vi "asdf.vi"(0 "ROI Descriptor (Image Mask 2)":T2={"Global Rectangle"=[63, 47, 555, 457], "Contours"=[{"ID"=enum."External", "Type"=3, "Coordinates"=[63, 47, 555, 457]}]} {"Contours"."Type" items=["No Selection", "Point", "Line", "Rectangle", "Oval", "Polygon", "Freehand Region", "Annulus", "Unused2", "Unused3", "Broken Line", "Freehand Line", "Rotated Rectangle"]}, 1 "Shrink (Image Mask 2)":bool=TRUE, 2 "Out / In (Image Mask 2)":bool, 3 "Color Plane (Color Plane Extraction 2)":i32(ring)=1 items=["Red", "Green", "Blue", "Hue", "Saturation", "Luminance", "Value", "Intensity"], 4 "Range (Threshold 3)":cluster{"Lower value":sgl, "Upper value":sgl}={"Lower value"=0.0, "Upper value"=222.0}, 5 "Operation (Gray Morphology 3)":T1(ring)=enum."Open", 6 "Structuring Element (Gray Morphology 3)":i32[][](array[numeric])=[[0, 1, 0], [1, 1, 1], [0, 1, 0]], 7 "error in":errorcluster, 8 "Min Radius (Circle Detection 2)":sgl=8.0, 9 "Max Radius (Circle Detection 2)":sgl=280.0) -> (20 "Nb Circles (Circle Detection 2)":i32, 21 "Circles Data (Circle Detection 2)":T4(array[cluster]), 22 "Circles Data (calibrated) (Circle Detection 2)":T4(array[cluster]), 27 "error out":errorcluster)   [LabVIEW 2018]
uses:
  <vilib>/vision/NI_Vision_Development_Module.lvlib
panel:
  out "Image Out":T3(plugin-control)
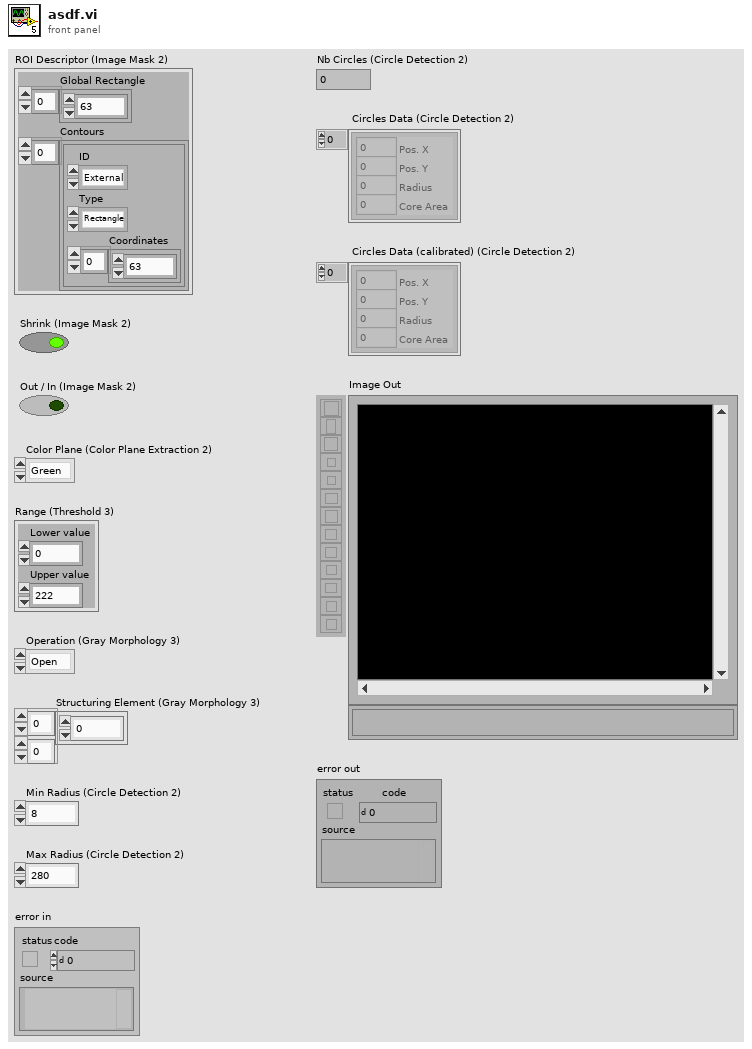
[diagram p1: front panel]
types:
  T1 = enum32{"AutoM", "Close", "Dilate", "Erode", "Gradient", "Gradient in", "Gradient out", "HitMiss", "Open", "PClose", "POpen", "Thick", "Thin"}
  T2 = cluster{"Global Rectangle":i32[], "Contours":cluster{"ID":enum32{"External", "Internal"}, "Type":u32, "Coordinates":i32[]}[]}
  T3 = typedef "IMAQ Image.ctl" = refnum<image>
  T4 = cluster{"Pos. X":i32, "Pos. Y":i32, "Radius":i32, "Core Area":i32}[]
  T5 = typedef "Image Type" = u32
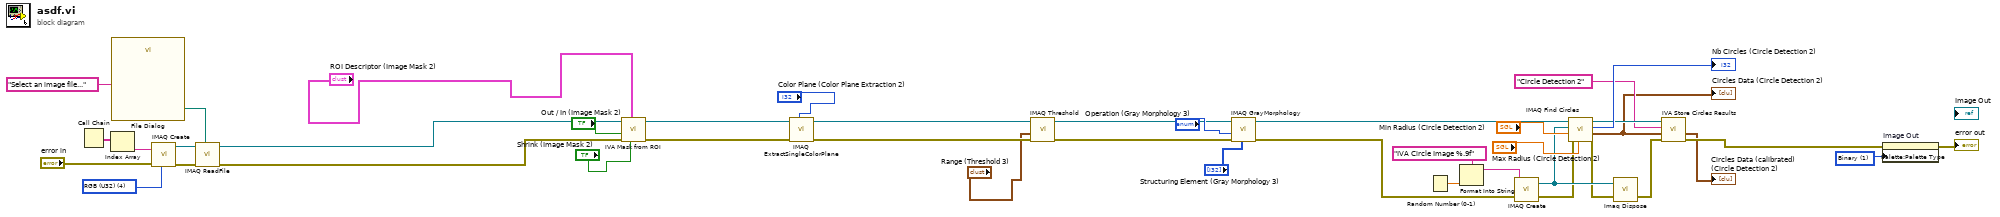
[diagram p0: block diagram]
diagram:
  w1 = u32 1 items=["Grayscale", "Binary", "Gradient", "Rainbow", "Temperature", "User Defined", "Binary 16 Bit", "Gradient 16 Bit", "Rainbow 16 Bit", "Temperature 16 Bit", "User Defined 16 Bit"] ("Palette Type")
  w33 = T5 4 items=["Grayscale (U8)", "Grayscale (I16)", "Grayscale (SGL)", "Complex (CSG)", "RGB (U32)", "HSL (U32)", "RGB (U64)", "Grayscale (U16)"] ("Image Type")
  n1 = Call Chain() -> (call chain=w37:string[])
  n2 = Index Array(array=w37) -> (element=w36:string)  [unwired: 1 in]
  n3 = call "File Dialog"("prompt"="Select an image file...") -> ("selected path"=w34:path)  [unwired: 6 in, 8 out]
  n4 = call "IMAQ Create"("Image Name"=w36, "Image Type"=w33, "error in (no error)"="error in") -> ("New Image"=w40:T3, "error out"=w39:errorcluster)  [unwired: 1 in, 1 out]
  n5 = call "IMAQ ReadFile"("File Path"=w34, "error in (no error)"=w39, "Image"=w40) -> ("error out"=w41:errorcluster, "Image Out"=w30:T3)  [unwired: 2 in, 5 out]
  n6 = call <vilib>:"IVA Mask from ROI.vi"("Shrink"="Shrink (Image Mask 2)", "ROI Descriptor"="ROI Descriptor (Image Mask 2)", "error in (no error)"=w41, "Out / In"="Out / In (Image Mask 2)", "Image Src"=w30) -> ("error out"=w28:errorcluster, "Image Out"=w26:T3)  [unwired: 5 out]
  n7 = call "IMAQ ExtractSingleColorPlane"("Color Plane"="Color Plane (Color Plane Extraction 2)", "error in (no error)"=w28, "Image Src"=w26) -> ("error out"=w25:errorcluster, "Image Dst Out"=w23:T3)  [unwired: 1 in, 6 out]
  n8 = call "IMAQ Threshold"("error in (no error)"=w25, "Range"="Range (Threshold 3)", "Image Src"=w23) -> ("error out"=w22:errorcluster, "Image Dst Out"=w19:T3)  [unwired: 3 in, 4 out]
  n9 = call "IMAQ GrayMorphology"("Structuring Element"="Structuring Element (Gray Morphology 3)", "error in (no error)"=w22, "Operation"="Operation (Gray Morphology 3)", "Image Src"=w19) -> ("error out"=w18:errorcluster, "Image Dst Out"=w9:T3)  [unwired: 3 in, 3 out]
  n10 = Random Number (0-1)() -> (number: 0 to 1=w3:dbl)
  n11 = Format Into String(format string="IVA Circle Image %.9f" ("Image Name"), w3) -> (resulting string=w5:string)  [unwired: 2 in, 1 out]
  n12 = call "IMAQ Create"("Image Name"=w5, "error in (no error)"=w18) -> ("New Image"=w14:T3, "error out"=w13:errorcluster)  [unwired: 2 in, 1 out]
  n13 = call "IMAQ Find Circles"("Max Radius"="Max Radius (Circle Detection 2)", "error in (no error)"=w13, "Min Radius"="Min Radius (Circle Detection 2)", "Image Dst"=w14, "Image Src"=w9) -> ("error out"=w12:errorcluster, "Circles Data"=w7:T4, "Nb Circles"=→"Nb Circles (Circle Detection 2)":i32)  [unwired: 4 out]
  "Circles Data (Circle Detection 2)" <- w7
  n14 = call "Imaq Dispose"("Image"=w14, "error in (no error)"=w12) -> ("error out"=w11:errorcluster)  [unwired: 1 in, 3 out]
  n15 = call <vilib>:"IVA Store Circles Results.vi"("error in (no error)"=w11, "Circles Data"=w7, "Step Name"="Circle Detection 2", "Image in"=w9) -> ("error out"=w10:errorcluster, "Circles Data (calibrated)"=→"Circles Data (calibrated) (Circle Detection 2)":T4)  [unwired: 6 out]
  n16 = property on="Image Out" class="ImageControl"(error in=w10, "Palette:Palette Type"=w1) -> (error out=→"error out":errorcluster)  [unwired: 1 in, 1 out]
